vi "convertTimestampToRaw.vi"(8 "error in (no error)":errorcluster, 10 "Timestamp":dbl format="%#.6g", 11 "Timestamp in":refnum<class "Timestamp.lvclass">) -> (0 "error out":errorcluster, 2 "Timestamp":u64, 3 "Timestamp out":refnum<class "Timestamp.lvclass">)   [LabVIEW 2016, in "RTTimestamp.lvlib" / "Timestamp.lvclass"]
uses:
  Timestamp.lvclass
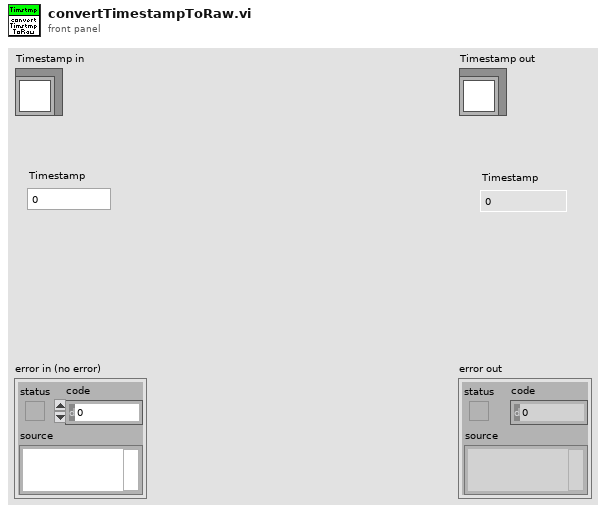
[diagram p1: front panel]
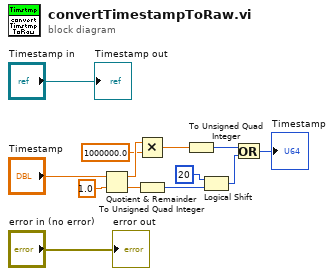
[diagram p0: block diagram]
diagram:
  n1 = Quotient & Remainder(x="Timestamp", y=1.0) -> (x-y*floor(x/y)=w9:dbl, floor(x/y)=w6:dbl)
  n2 = Multiply(x=w9, y=1000000.0) -> (x*y=w7:dbl)
  n3 = To Unsigned Quad Integer(1:w6) -> (0:w5:u64)
  n4 = To Unsigned Quad Integer(1:w7) -> (0:w3:u64)
  n5 = Logical Shift(y=i16 20, x=w5) -> (x << y=w2:u64)
  n6 = Or(x=w3, y=w2) -> (x .or. y?=→"Timestamp":u64)
  "error out" <- "error in (no error)"
  "Timestamp out" <- "Timestamp in"
